vi "Get CArm Angle and Height.vi"(8 "error in (no error)":errorcluster, 11 "XRay CArm in":refnum<class "XRay CArm.lvclass">) -> (0 "error out":errorcluster, 1 "CArm Height":sgl, 2 "CArm Angle":sgl, 3 "XRay CArm out":refnum<class "XRay CArm.lvclass">, 5 "Pos Changed":bool)   [LabVIEW 2026, in "XRay CArm.lvclass"]
uses:
  XRay CArm.lvclass
  XRay CArm.lvclass/XRay CArm.ctl
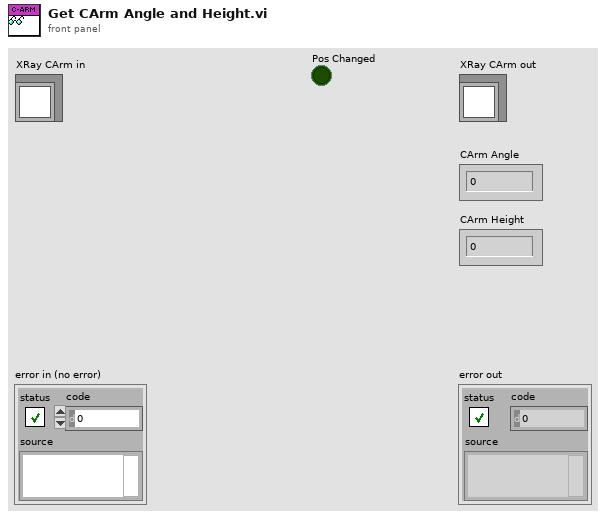
[diagram p1: front panel]
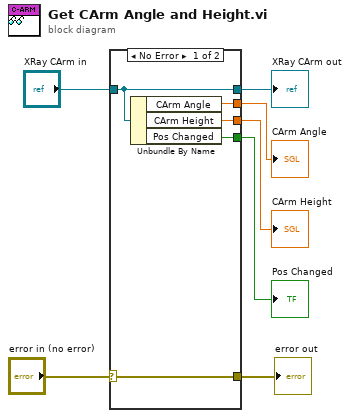
[diagram p0: block diagram]
diagram:
  n1 = case shown="No Error" "error in (no error)" {
    selector: "error in (no error)" -> [w12 w13]
    tunnel: [w12 w13] -> w6
    tunnel: [w11 w14] -> w4
    tunnel: "XRay CArm in" -> [w11 w14]
    tunnel: [w10 _] -> w3
    tunnel: [w9 _] -> w2
    tunnel: [w8 _] -> w1
    frame No Error {
      n2 = Unbundle By Name(w11) -> ("CArm Angle"=w10:sgl, "CArm Height"=w9:sgl, "Pos Changed"=w8:bool)
    }
    frame Error {
    }
  }
  "error out" <- w6
  "XRay CArm out" <- w4
  "CArm Angle" <- w3
  "CArm Height" <- w2
  "Pos Changed" <- w1
